vi "movable.vi"(0 "i1":i32, 1 "j1":i32, 2 "i2":i32, 3 "j2":i32, 4 "turn":i32) -> (5 "valid":bool)   [LabVIEW 2024]
uses:
  globalVar.vi
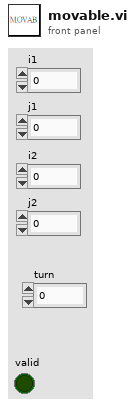
[diagram p1: front panel]
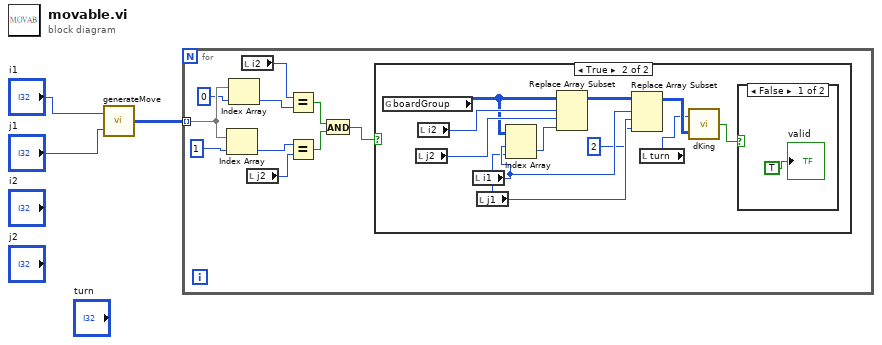
[diagram p0: block diagram]
diagram:
  n1 = call "generateMove.vi"("j"="j1", "i"="i1") -> ("Array"=w1:i32[][])
  n2 = for {
    tunnel: w1 -> [w13] mode=indexing
    n3 = Index Array(array=w13, index=1) -> (element=w8:i32)
    n4 = Index Array(array=w13, index=0) -> (element=w10:i32)
    n5 = local read "i2"() -> (w9:i32)
    n6 = local read "j2"() -> (w7:i32)
    n7 = Equal?(x=w9, y=w10) -> (x = y?=w6:bool)
    n8 = Equal?(x=w8, y=w7) -> (x = y?=w5:bool)
    n9 = And(x=w6, y=w5) -> (x .and. y?=w4:bool)
    n10 = case shown="True" w4 {
      frame False {
      }
      frame True {
        n11 = global read "globalVar.vi" "boardGroup"() -> (w21:i32[][])
        n12 = local read "j2"() -> (w23:i32)
        n13 = local read "i2"() -> (w24:i32)
        n14 = local read "i1"() -> (w19:i32)
        n15 = local read "j1"() -> (w18:i32)
        n16 = Index Array(array=w21, index (row)=w19, index (col)=w18) -> (element=w22:i32)
        n17 = Replace Array Subset(array=w21, new element=w22, index (row)=w24, index (col)=w23) -> (w20:i32[][])
        n18 = Replace Array Subset(array=w20, new element=2 ("new element/subarray"), index (row)=w19, index (col)=w18) -> (w16:i32[][])
        n19 = local read "turn"() -> (w15:i32)
        n20 = call "dKing.vi"("boardGroup"=w16, "turn"=w15) -> ("isDKing"=w14:bool)
        n21 = case shown="False" w14 {
          frame False {
            "valid" <- TRUE ("valid")
          }
          frame True {
          }
        }
      }
    }
  }
